vi "多路停止(FGStop).vi"(0 "error in (no error)":errorcluster caption="错误输入（无错误）", 2 "停止1":bool, 3 "停止":bool, 4 "停止2":bool) -> (7 "error in (no error)":errorcluster caption="错误输入（无错误）", 10 "Output":bool)   [LabVIEW 2012]
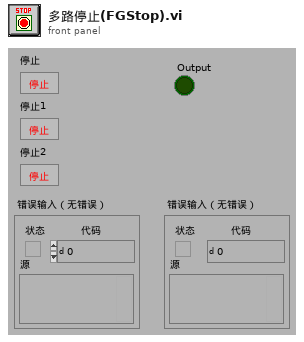
[diagram p1: front panel]
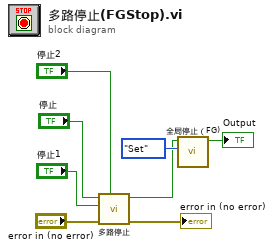
[diagram p0: block diagram]
diagram:
  n1 = call "多路停止.vi"("error in (no error)"="error in (no error)", "停止1"="停止1", "停止"="停止", "停止2"="停止2") -> ("error in (no error)"=→"error in (no error)":errorcluster, "为真停止"=w2:bool)  [unwired: 4 in, 1 out]
  n2 = call "全局停止（FG).vi"("Mode"=enum16{"Init", "Set", "Get"}."Set", "Input"=w2) -> ("Output"=→"Output":bool)  [unwired: 8 in, 1 out]
